vi "Return to Thread Pool.vi"(8 "error in (no error)":errorcluster, 10 "Transfer Group in":refnum<class "Transfer Group.lvclass">, 11 "Plugin Thread in":refnum<class "Plugin Thread.lvclass">) -> (0 "error out":errorcluster, 3 "Plugin Thread out":refnum<class "Plugin Thread.lvclass">)   [LabVIEW 2017, in "DSF Core.lvlib" / "Plugin Thread.lvclass"]
uses:
  Thread/Plugin/Plugin Thread.lvclass
  Transfer Group/Transfer Group.lvclass
  Transfer Group/Transfer Group.lvclass/Transfer Group.ctl
  Thread/Plugin/Plugin Thread.lvclass/Plugin Thread.ctl
  Interfaces/Interface/Interface.lvclass/Interface.ctl
  Thread Pool/Pool.lvclass/Pool.ctl
  Thread Pool/Write FIFO.vi
  Interfaces/Interface/Get ID.vi
  Interfaces/Transceiver Interface/Plugin Interface.lvclass
  C:/Users/Admin/Desktop/Data Sharing Framework/Source/Core/Engine/Classes/Interfaces/Interface/Interface.lvclass
  Thread Pool/Plugin Interface Pool.lvclass
  C:/Users/Admin/Desktop/Data Sharing Framework/Source/Core/Engine/Classes/Thread Pool/Pool.lvclass
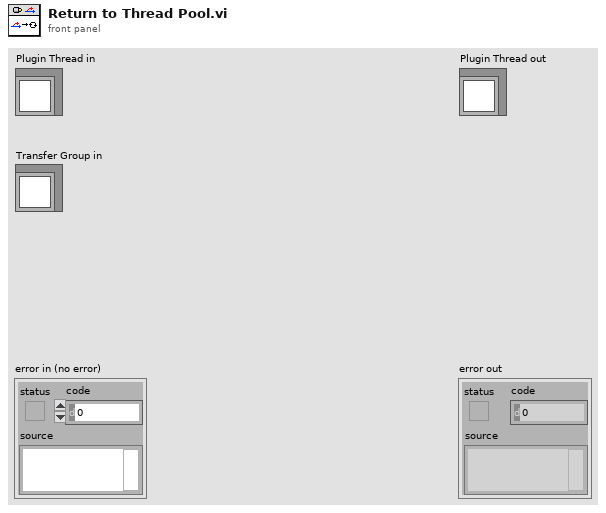
[diagram p1: front panel]
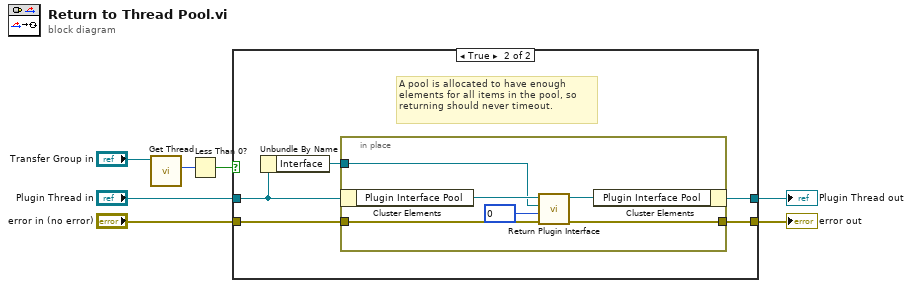
[diagram p0: block diagram]
diagram:
  n1 = call "Get Thread.vi"("Transfer Group in"="Transfer Group in") -> ("thread"=w2:i32)  [unwired: 9 in, 1 out]
  n2 = Less Than 0?(x=w2) -> (x < 0?=w1:bool)
  n3 = case shown="True" w1 {
    tunnel: "error in (no error)" -> [w8 w14]
    tunnel: [w8 w13] -> w6
    tunnel: "Plugin Thread in" -> [w9 w12]
    tunnel: [w9 w10] -> w4
    frame False {
      # "Thread is 0 or greater, meaning this thread was manually dispatched to, so don't return to thread pool."
    }
    frame True {
      # "A pool is allocated to have enough elements for all items in the pool, so returning should never timeout."
      n4 = Unbundle By Name(w12) -> ("Interface"=w11:refnum<class "Plugin Interface.lvclass">)
      n5 = in-place {
        in-place-border: w14 -> [w20]
        in-place-border: [w19] -> w13
        in-place-border: w11 -> [w16]
        n6 = in-place-cluster #1(w12) -> ("Plugin Interface Pool"=w18:refnum<class "Plugin Interface Pool.lvclass">)
        n7 = call "Return Plugin Interface.vi"("error in (no error)"=w20, "timeout in ms (0)"=0, "Plugin Interface"=w16, "Plugin Interface Pool in"=w18) -> ("error out"=w19:errorcluster, "Plugin Interface Pool out"=w17:refnum<class "Plugin Interface Pool.lvclass">)  [unwired: 5 in, 1 out]
        n8 = in-place-cluster #1("Plugin Interface Pool"=w17) -> (w10:refnum<class "Plugin Thread.lvclass">)
      }
    }
  }
  "error out" <- w6
  "Plugin Thread out" <- w4
